vi "getClaseProducto.vi"(0 "claseProducto.lvclass":refnum<class "claseProducto.lvclass">, 3 "error in":errorcluster) -> (7 "claseProducto.lvclass 2":refnum<class "claseProducto.lvclass">, 8 "dataReading":T1, 10 "error out":errorcluster)   [LabVIEW 2014, in "claseProducto.lvclass"]
uses:
  claseProducto.lvclass
  claseProducto.lvclass/claseProducto.ctl
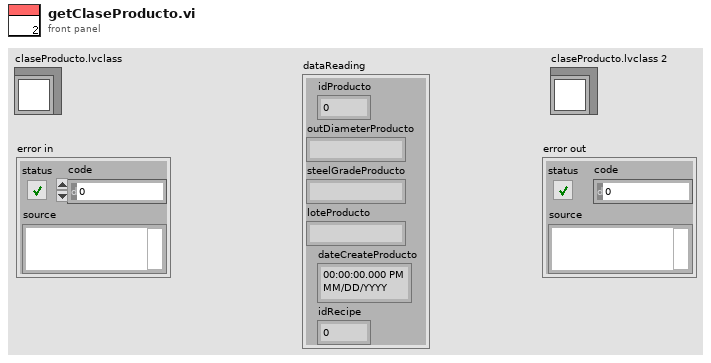
[diagram p1: front panel]
types:
  T1 = cluster{"idProducto":dbl, "outDiameterProducto":string, "steelGradeProducto":string, "loteProducto":string, "dateCreateProducto":timestamp, "idRecipe":dbl}
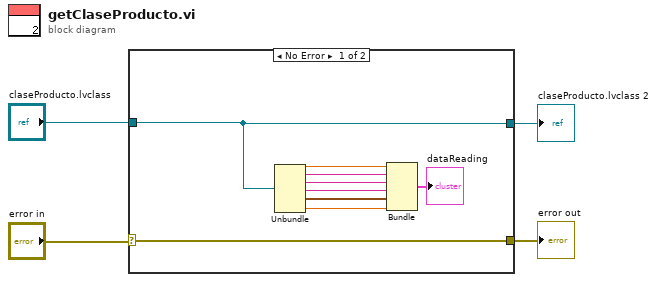
[diagram p0: block diagram]
diagram:
  n1 = case shown="No Error" "error in" {
    selector: "error in" -> [w13 w15]
    tunnel: [w13 w15] -> w3
    tunnel: "claseProducto.lvclass" -> [w12 w14]
    tunnel: [w12 w14] -> w1
    frame No Error {
      n2 = Unbundle(w12) -> (w11:dbl, w10:string, w9:string, w8:string, w7:timestamp, w6:dbl)
      n3 = Bundle("idProducto"=w11, "outDiameterProducto"=w10, "steelGradeProducto"=w9, "loteProducto"=w8, "dateCreateProducto"=w7, "idRecipe"=w6) -> (→"dataReading":T1)  [unwired: 1 in]
    }
    frame Error {
    }
  }
  "claseProducto.lvclass 2" <- w1
  "error out" <- w3
